vi "Untitled 1.vi"() -> ()   [LabVIEW 2024]
uses:
  <vilib>/measure/maspectr.llb/Power Spectrum and PSD Export Mode.ctl
  <vilib>/measure/maspectr.llb/FFT Power Spectrum and PSD for 1 Chan.vi
  <vilib>/measure/NI_MABase.lvlib
  <vilib>/measure/NI_MAPro.lvlib
panel:
  out "x/y":dbl
  out "Waveform Graph":cluster{"f0":dbl, "df":dbl, "magnitude":dbl[]}(graph)
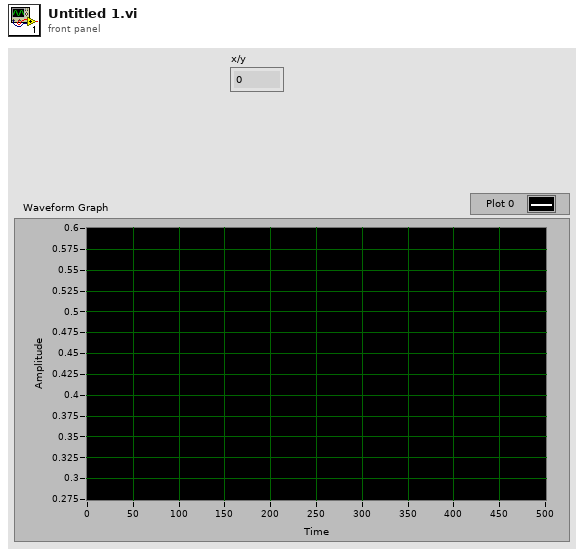
[diagram p1: front panel]
types:
  T1 = cluster{"averaging mode":enum16{"No averaging", "Vector averaging", "RMS averaging", "Peak hold"}, "weighting mode":enum16{"Linear", "Exponential"}, "number of averages":u32}
  T2 = typedef "NI_MAPro.lvlib/Power Spectrum and PSD Export Mode.ctl" = u16
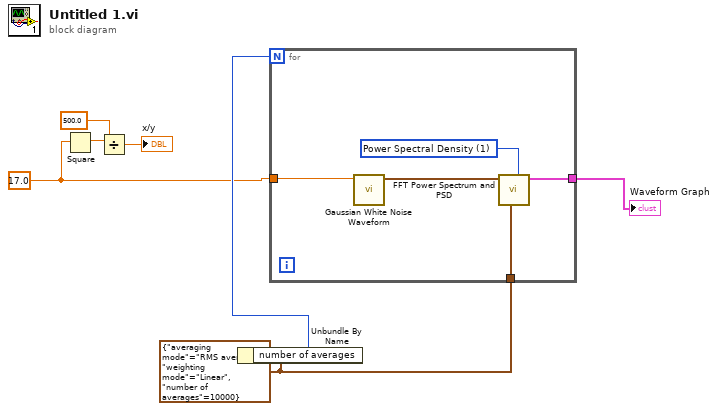
[diagram p0: block diagram]
diagram:
  w6 = T1 {"averaging mode"=enum."RMS averaging", "weighting mode"=enum."Linear", "number of averages"=10000} ("averaging parameters")
  w4 = 17.0 ("standard deviation")
  n1 = Square(x=w4) -> (x^2=w3:dbl)
  n2 = Divide(x=w3, y=500.0) -> (x/y=→"x/y":dbl)
  n3 = Unbundle By Name(w6) -> ("number of averages"=w5:u32)
  n4 = for {
    N: w5 -> [_]
    tunnel: w4 -> [w12]
    tunnel: [w10] -> w7
    tunnel: w6 -> [w9]
    w8 = T2 1 items=["Power Spectrum", "Power Spectral Density"] ("export mode")
    n5 = call <vilib>:"Gaussian White Noise Waveform.vi"("standard deviation"=w12) -> ("signal out"=w11:waveform(dbl))  [unwired: 9 in, 1 out]
    n6 = call-poly <vilib>:"FFT Power Spectrum and PSD.vi"("export mode"=w8, "averaging parameters"=w9, "time signal"=w11) -> ("Power Spectrum / PSD"=w10:cluster{"f0":dbl, "df":dbl, "magnitude":dbl[]})  [unwired: 5 in, 3 out]
  }
  "Waveform Graph" <- w7
